vi "ValidateStringRegExp.vi"(9 "Pattern In":string, 11 "String To Match":string) -> (1 "Match Found":bool, 3 "String Out":string)   [LabVIEW 2026]
uses:
  <vilib>/regexp/Match Regular Expression.xnode
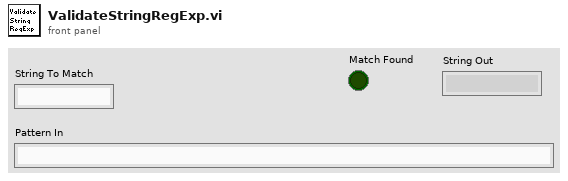
[diagram p1: front panel]
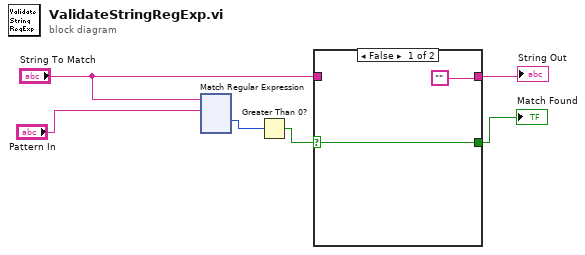
[diagram p0: block diagram]
diagram:
  n1 = xnode "Match Regular Expression"("input string"="String To Match", "regular expression"="Pattern In") -> ("offset past match"=w5:i32)  [unwired: 4 in, 4 out]
  n2 = Greater Than 0?(x=w5) -> (x > 0?=w6:bool)
  n3 = case shown="False" w6 {
    selector: w6 -> [w8 w9]
    tunnel: "String To Match" -> [_ w10]
    tunnel: ["" w10] -> w2
    tunnel: [w8 w9] -> w1
    frame False {
    }
    frame True {
    }
  }
  "String Out" <- w2
  "Match Found" <- w1
